vi "Cell Enable All.vi"(7 "Box ID":u8=1, 8 "error in (no error)":errorcluster, 10 "Enable":bool, 11 "CAN in":refnum<class "XNET_BS120x.lvclass">) -> (0 "error out":errorcluster, 3 "CAN out":refnum<class "XNET_BS120x.lvclass">)   [LabVIEW 2021, in "BS120x Driver.lvlib" / "XNET_BS120x.lvclass"]
uses:
  XNET_BS120x.lvclass
  BS120x.lvclass
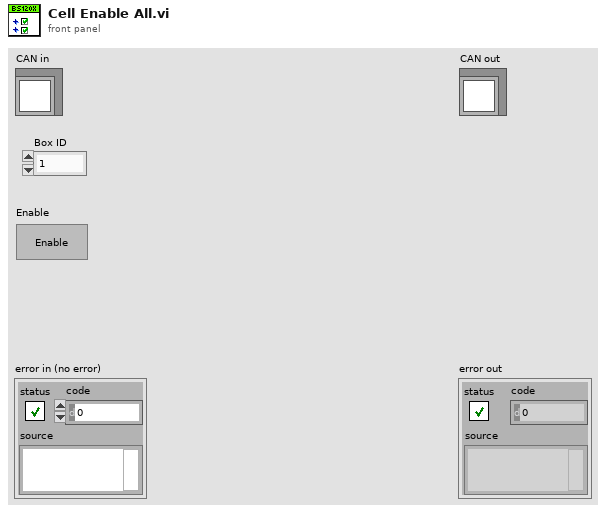
[diagram p1: front panel]
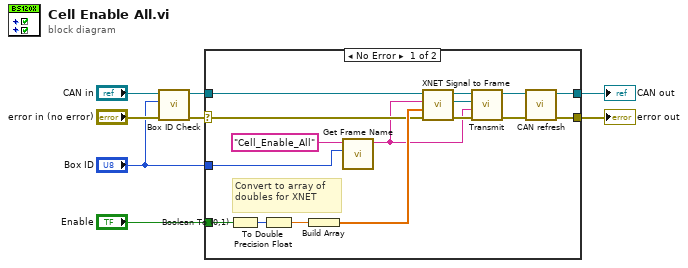
[diagram p0: block diagram]
diagram:
  n1 = call "Box ID Check.vi"("error in (no error)"="error in (no error)", "Box ID"="Box ID", "CAN in"="CAN in") -> ("error out"=w1:errorcluster, "CAN out"=w4:refnum<class "XNET_BS120x.lvclass">)  [unwired: 7 in]
  n2 = case shown="No Error" w1 {
    selector: w1 -> [w10 w26]
    tunnel: "Enable" -> [w21 _]
    tunnel: w4 -> [w19 w25]
    tunnel: [w15 w26] -> w6
    tunnel: [w13 w25] -> w5
    tunnel: "Box ID" -> [w11 _]
    frame No Error {
      # "Convert to array of doubles for XNET"
      n3 = Boolean To (0,1)(Boolean=w21) -> (0, 1=w23:i16)
      n4 = To Double Precision Float(number=w23) -> (double precision float=w24:dbl)
      n5 = Build Array(w24) -> (w20:dbl[])
      n6 = call "Get Frame Name.vi"("Box ID"=w11, "Frame Name"="Cell_Enable_All" ("Frame")) -> ("Frame Name out"=w9:string)  [unwired: 9 in]
      n7 = call "XNET Signal to Frame.vi"("error in (no error)"=w10, "Data Array"=w20, "Frame"=w9, "CAN in"=w19) -> ("error out"=w22:errorcluster, "Data"=w17:refnum<class "XNET Data.lvclass">, "CAN out"=w18:refnum<class "XNET_BS120x.lvclass">)  [unwired: 5 in]
      n8 = call "Transmit.vi"("error in (no error)"=w22, "Frame"=w9, "Data in"=w17, "CAN in"=w18) -> ("error out"=w16:errorcluster, "CAN out"=w14:refnum<class "XNET_BS120x.lvclass">)  [unwired: 6 in]
      n9 = call "CAN refresh.vi"("error in (no error)"=w16, "CAN in"=w14) -> ("error out"=w15:errorcluster, "CAN out"=w13:refnum<class "XNET_BS120x.lvclass">)  [unwired: 8 in]
    }
    frame Error {
    }
  }
  "error out" <- w6
  "CAN out" <- w5
